vi "ControlPID_SeguidorLuz_2GL.vi"() -> ()   [LabVIEW 2015]
uses:
  <vilib>/MakerHub/LINX/Public/Peripherals/Digital/Digital Write N Chans.vi
  <vilib>/MakerHub/LINX/Public/Peripherals/Analog/Analog Read N Chans.vi
  <vilib>/MakerHub/LINX/Private/Local IO/LinxDigitalWrite.vi
  <vilib>/MakerHub/LINX/Public/Utilities/Check Channel.vi
  <vilib>/MakerHub/LINX/Private/Local IO/LinxAnalogRead.vi
  <vilib>/MakerHub/LINX/Public/Utilities/Open Serial.vi
  <vilib>/MakerHub/LINX/Private/Utilties/Generate Error.vi
  <vilib>/MakerHub/LINX/Public/Peripherals/PWM/PWM Set Duty Cycle N Chans.vi
  <vilib>/MakerHub/LINX/LMH-LINX.lvlib
  <vilib>/MakerHub/LINX/Public/Sensors/Distance/Ultrasonic/Ultrasonic.lvlib
panel:
  in  "Ajuste de\nTemp. °C":i32(slide)=63 scale=0.0..100.0
  out "Sistema \nActivo":bool
  out "PWM\nBase":dbl
  out "PWM\nPanel":dbl
  in  "Kp 2":dbl=1.5
  in  "Ki 2":dbl=0.001
  in  "Kd 2":dbl=0.001
  in  "Kd 1":dbl=0.001
  in  "Ki 1":dbl=0.001
  in  "Kp 1":dbl=1.0
  out "S. Luz 4":dbl format="%#_4g"
  out "S. Luz 3":dbl format="%#_4g"
  out "S. Luz 2":dbl format="%#_4g"
  out "S. Luz 1":dbl format="%#_4g"
  out "Bajo\nNivel":bool
  out "Baja\nTemp.":bool
  out "Temperatura °C":dbl(slide) scale=0.0..100.0
  out "Temperaturas °C":dbl[](array[numeric])=[29.0]
  out "Tanque L":dbl(slide) scale=0.0..1.0
  in  "Pausa":bool
  in  "Arranque":bool
  in  "Paro":bool
  out "Dispositivo conectado":string
  in  "Puerto":refnum<visa-resource-name>="COM3"
  # "Universidad Nacional Autónoma de México\nFacultad de Ingeniería\nLab. De Instrumentación Virtual\n\nProyecto Final: Calentador de agua mediante un seguidor solar"
  # "Configuración PID"
  # "Supervisión de sistema"
  # "Control de programa"
  # "Motor\nPanel"
  # "Motor\nBase"
  # "Saturación\nSensores"
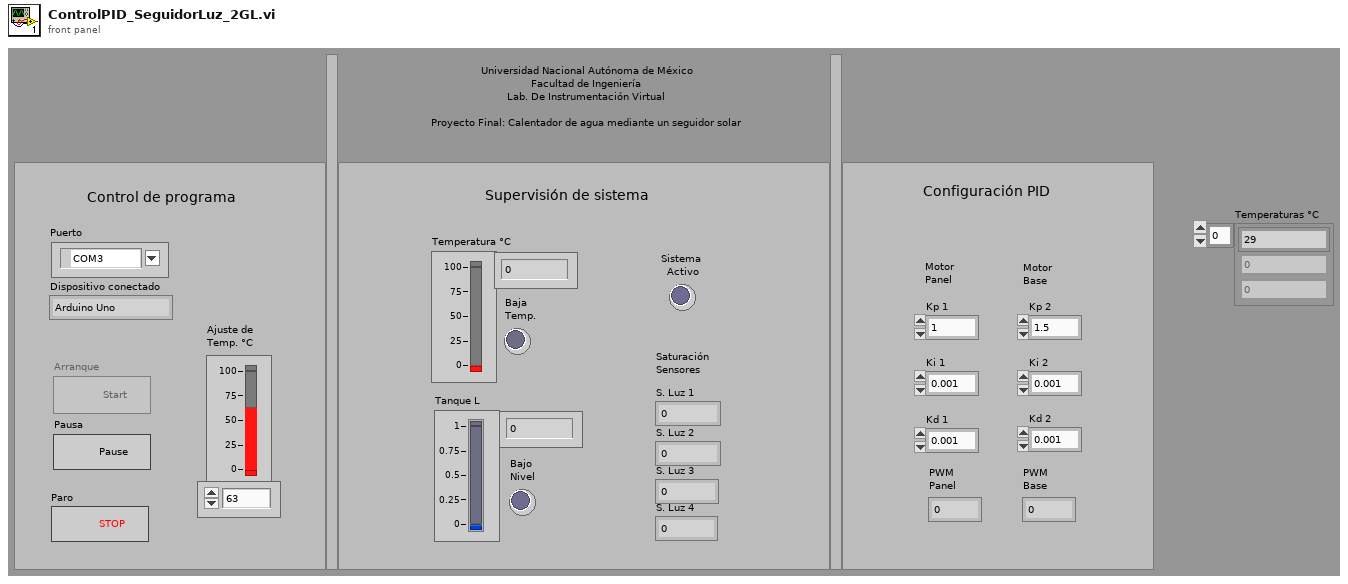
[diagram p1: front panel]
types:
  T1 = enum8{"Enabled", "Disabled", "Disabled and Grayed Out"}
  T2 = enum16{"Espera", "Nivel_Temp", "Reposo", "PID", "Fin"}
  T3 = typedef "LMH-LINX.lvlib/LINX Ref.ctl" = cluster{"IO":T4, "Interface":T5, "LINX Device Config":T6}
  T4 = typedef "LMH-LINX.lvlib/Platform.ctl" = enum16{"Remote", "Local"}
  T5 = typedef "LMH-LINX.lvlib/Interface.ctl" = enum16{"Serial", "TCP"}
  T6 = typedef "LMH-LINX.lvlib/Device.lvlib/LINX Device Config.ctl" = cluster{"Interface":T5, "COM Port":refnum<visa-resource-name>, "TCP Configuration":T7, "Device Family":u8, "Device ID":u8, "Device Name":string, "TCP Ref":refnum<k5>, "Channels":T8}
  T7 = typedef "LMH-LINX.lvlib/Device.lvlib/TCP Config.ctl" = cluster{"IP Address":string, "Port":u16}
  T8 = typedef "LMH-LINX.lvlib/Channels.ctl" = cluster{"DI":u8[], "DO":u8[], "AI":u8[], "AO":u8[], "PWM":u8[], "QE":u8[], "UART":u8[], "I2C 2":u8[], "SPI":u8[], "CAN":u8[], "Servo":u8[], "AI Ref (V)":dbl, "AI Resolution (Bits)":u8, "AO Ref (V)":dbl, "AO Resolution (Bits)":u8}
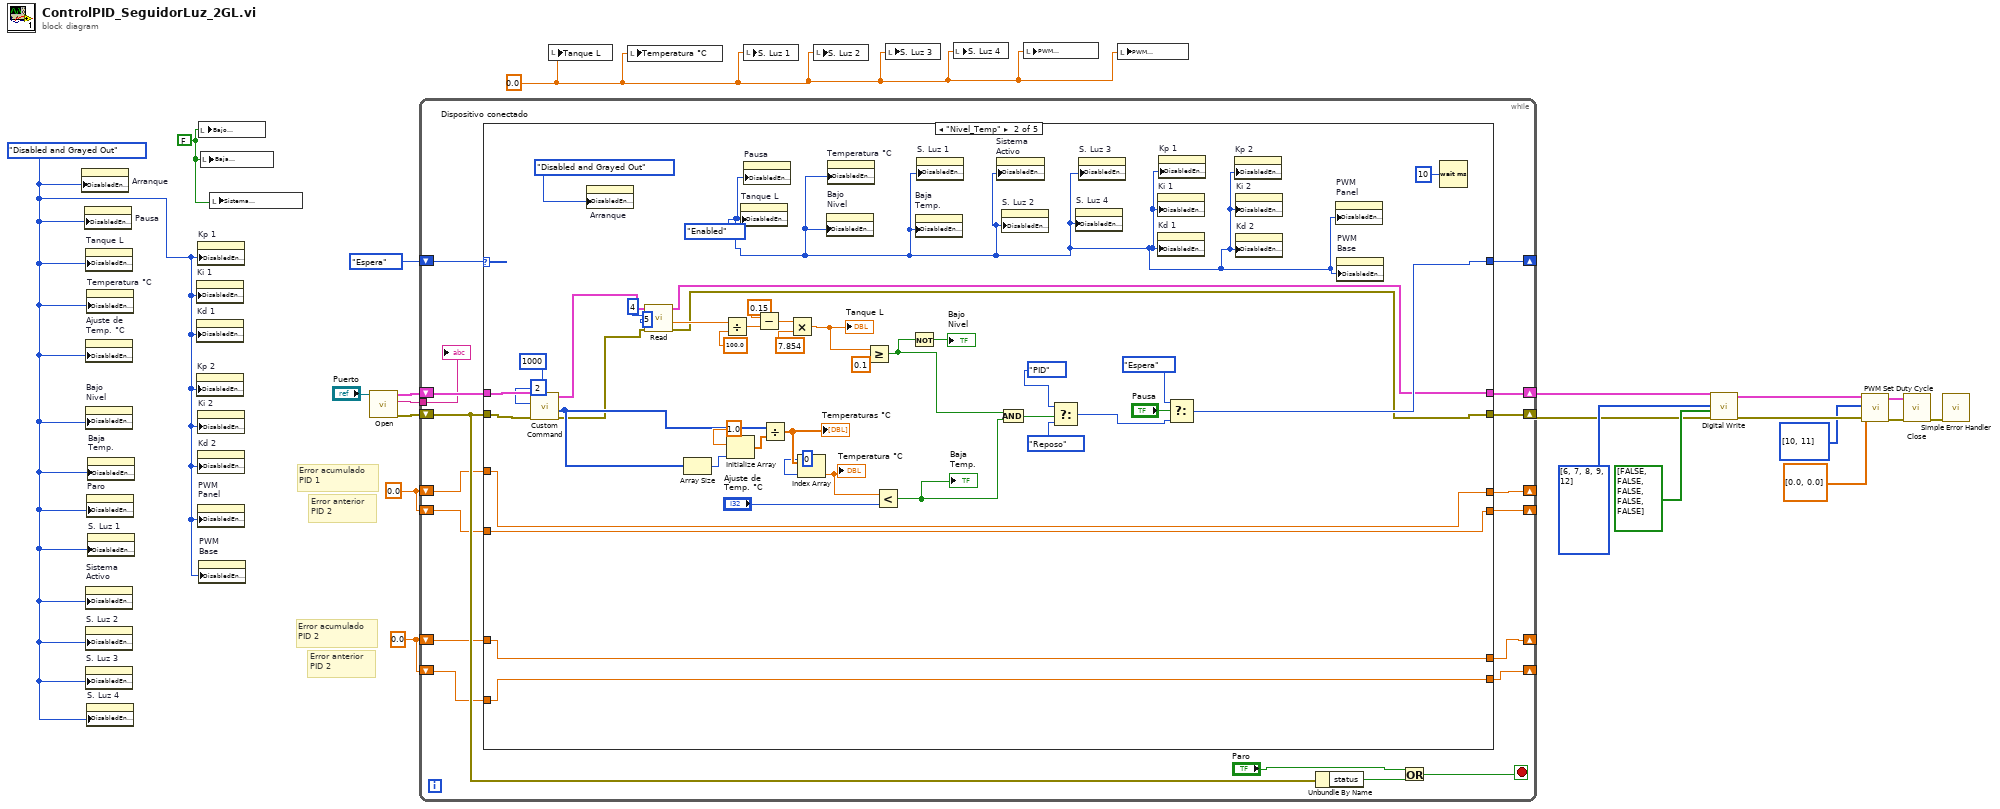
[diagram p0: block diagram]
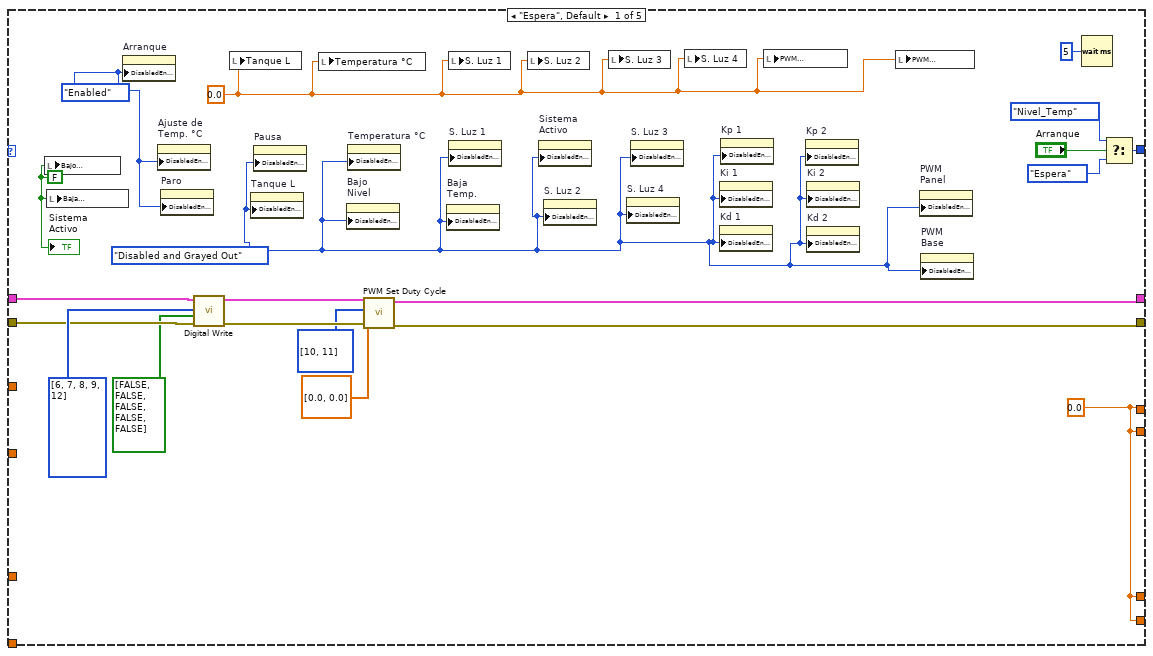
[diagram p2: hidden frame]
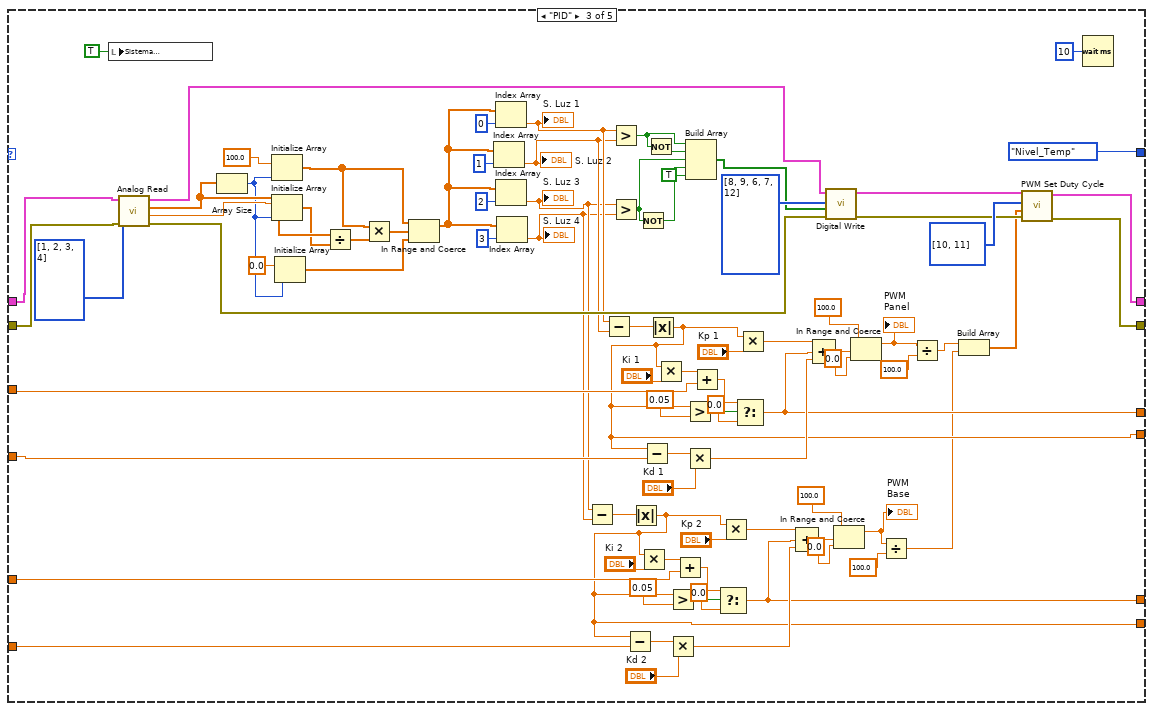
[diagram p3: hidden frame]
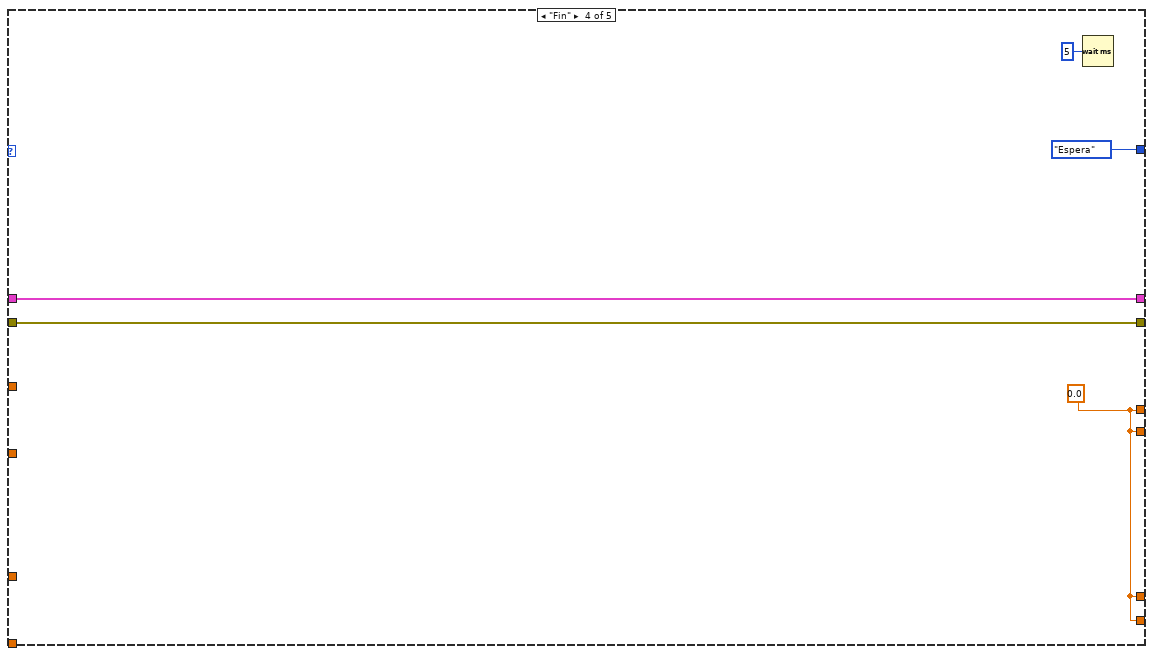
[diagram p4: hidden frame]
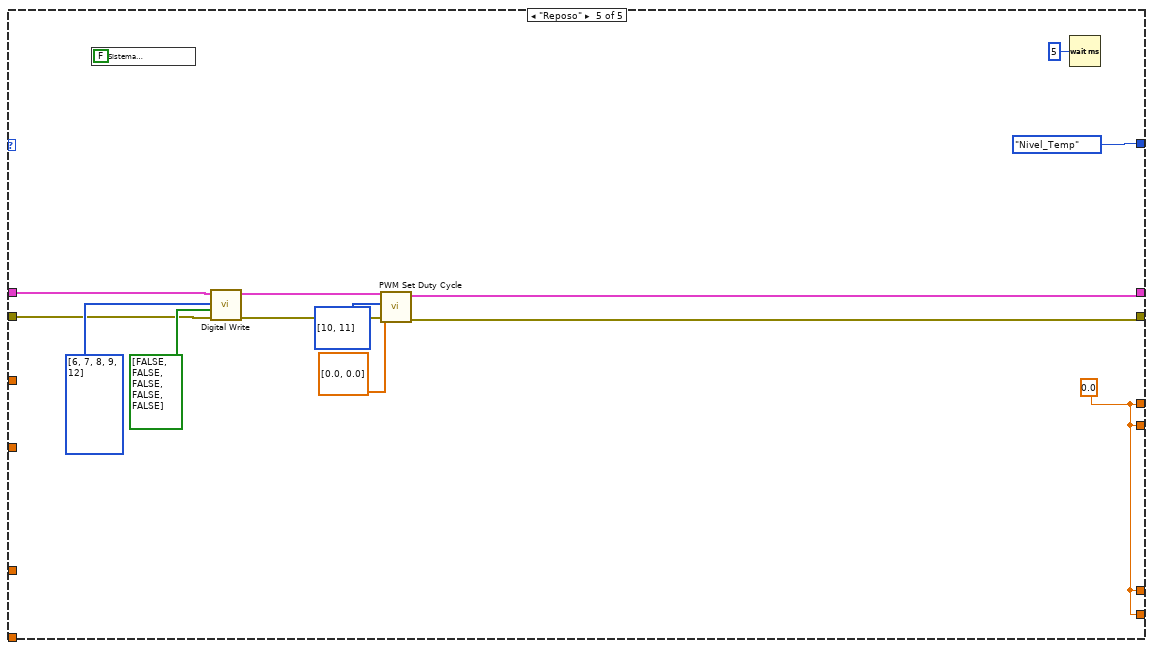
[diagram p5: hidden frame]
diagram:
  w11 = FALSE ("Bajo\nNivel")
  w13 = 0.0 ("Tanque L")
  w14 = 0.0
  w15 = 0.0
  w12 = T1."Disabled and Grayed Out" ("Disabled")
  # "Error anterior \nPID 2"
  # "Error acumulado\nPID 2"
  # "Error anterior \nPID 2"
  # "Error acumulado\nPID 1"
  n1 = property on="Arranque" class="Bool (strict)"("DisabledEnum"=w12) -> ()  [unwired: 2 in, 2 out]
  n2 = property on="Pausa" class="Bool (strict)"("DisabledEnum"=w12) -> ()  [unwired: 2 in, 2 out]
  n3 = property on="Tanque L" class="Slide (strict)"("DisabledEnum"=w12) -> ()  [unwired: 2 in, 2 out]
  n4 = property on="Ajuste de\nTemp. °C" class="Slide (strict)"("DisabledEnum"=w12) -> ()  [unwired: 2 in, 2 out]
  n5 = property on="Bajo\nNivel" class="Bool (strict)"("DisabledEnum"=w12) -> ()  [unwired: 2 in, 2 out]
  n6 = property on="Sistema \nActivo" class="Bool (strict)"("DisabledEnum"=w12) -> ()  [unwired: 2 in, 2 out]
  n7 = property on="S. Luz 2" class="DigNum (strict)"("DisabledEnum"=w12) -> ()  [unwired: 2 in, 2 out]
  n8 = property on="S. Luz 3" class="DigNum (strict)"("DisabledEnum"=w12) -> ()  [unwired: 2 in, 2 out]
  n9 = property on="Temperatura °C" class="Slide (strict)"("DisabledEnum"=w12) -> ()  [unwired: 2 in, 2 out]
  n10 = property on="Paro" class="Bool"("DisabledEnum"=w12) -> ()  [unwired: 2 in, 2 out]
  n11 = property on="S. Luz 4" class="DigNum (strict)"("DisabledEnum"=w12) -> ()  [unwired: 2 in, 2 out]
  n12 = property on="Baja\nTemp." class="Bool (strict)"("DisabledEnum"=w12) -> ()  [unwired: 2 in, 2 out]
  n13 = property on="S. Luz 1" class="DigNum (strict)"("DisabledEnum"=w12) -> ()  [unwired: 2 in, 2 out]
  n14 = property on="Ki 1" class="DigNum (strict)"("DisabledEnum"=w12) -> ()  [unwired: 2 in, 2 out]
  n15 = property on="Kd 1" class="DigNum (strict)"("DisabledEnum"=w12) -> ()  [unwired: 2 in, 2 out]
  n16 = property on="Kp 2" class="DigNum (strict)"("DisabledEnum"=w12) -> ()  [unwired: 2 in, 2 out]
  n17 = property on="Kp 1" class="DigNum (strict)"("DisabledEnum"=w12) -> ()  [unwired: 2 in, 2 out]
  n18 = property on="Ki 2" class="DigNum (strict)"("DisabledEnum"=w12) -> ()  [unwired: 2 in, 2 out]
  n19 = property on="Kd 2" class="DigNum (strict)"("DisabledEnum"=w12) -> ()  [unwired: 2 in, 2 out]
  n20 = property on="PWM\nPanel" class="DigNum (strict)"("DisabledEnum"=w12) -> ()  [unwired: 2 in, 2 out]
  n21 = local write "Bajo\nNivel"(w11) -> ()
  n22 = property on="PWM\nBase" class="DigNum (strict)"("DisabledEnum"=w12) -> ()  [unwired: 2 in, 2 out]
  n23 = local write "Baja\nTemp."(w11) -> ()
  n24 = local write "Sistema \nActivo"(w11) -> ()
  n25 = call-poly <vilib>:"Open.vi"("Serial Port"="Puerto") -> ("Error Out"=w17:errorcluster, "Device Name"=w18:string, "LINX Resource"=w19:T3)  [unwired: 8 in]
  n26 = while {
    shift-right: [w36] -> _
    shift-left: T2."Espera" -> [w39]
    tunnel: w18 -> [w37]
    shift-right: [w35] -> w2
    shift-left: w19 -> [w38]
    shift-right: [w34] -> w1
    shift-left: w17 -> [w33]
    shift-right: [w27] -> _
    shift-left: w15 -> [w29]
    shift-right: [w26] -> _
    shift-left: w15 -> [w28]
    shift-right: [w23] -> _
    shift-left: w14 -> [w25]
    shift-right: [w22] -> _
    shift-left: w14 -> [w24]
    stop <- w30 stop-if-true
    n27 = case shown="\"Nivel_Temp\"" w39 {
      tunnel: w38 -> [w54 w99 w141 w190 w199]
      tunnel: w33 -> [w53 w98 w140 w189 w198]
      tunnel: [w56 w74 T2."Nivel_Temp" T2."Espera" T2."Nivel_Temp"] -> w36
      tunnel: [w47 w68 w143 w190 w197] -> w35
      tunnel: [w46 w67 w142 w189 w196] -> w34
      tunnel: w29 -> [_ w66 w150 _ _]
      tunnel: w28 -> [_ w65 w144 _ _]
      tunnel: [w44 w66 w133 w187 w193] -> w27
      tunnel: [w44 w65 w132 w187 w193] -> w26
      tunnel: w25 -> [_ w64 w114 _ _]
      tunnel: w24 -> [_ w63 w113 _ _]
      tunnel: [w44 w64 w112 w187 w193] -> w23
      tunnel: [w44 w63 w111 w187 w193] -> w22
      frame "Espera", Default {
        w40 = T1."Disabled and Grayed Out" ("Disabled")
        w42 = 0.0 ("Tanque L")
        w43 = FALSE ("Bajo\nNivel")
        w44 = 0.0
        w41 = T1."Enabled" ("Disabled")
        n28 = local write "Bajo\nNivel"(w43) -> ()
        n29 = local write "Baja\nTemp."(w43) -> ()
        n30 = property on="Arranque" class="Bool (strict)"("DisabledEnum"=w41) -> ()  [unwired: 2 in, 2 out]
        n31 = property on="Ajuste de\nTemp. °C" class="Slide (strict)"("DisabledEnum"=w41) -> ()  [unwired: 2 in, 2 out]
        n32 = property on="Paro" class="Bool"("DisabledEnum"=w41) -> ()  [unwired: 2 in, 2 out]
        n33 = call-poly <vilib>:"Digital Write.vi"("Error In"=w53, "Values"=bool[] [FALSE, FALSE, FALSE, FALSE, FALSE], "DO Channels"=u8[] [6, 7, 8, 9, 12], "LINX Resource"=w54) -> ("Error Out"=w51:errorcluster, "LINX Resource"=w52:T3)  [unwired: 6 in]
        n34 = local write "Tanque L"(w42) -> ()
        n35 = property on="Tanque L" class="Slide (strict)"("DisabledEnum"=w40) -> ()  [unwired: 2 in, 2 out]
        n36 = property on="Pausa" class="Bool (strict)"("DisabledEnum"=w40) -> ()  [unwired: 2 in, 2 out]
        n37 = local write "Temperatura °C"(w42) -> ()
        n38 = property on="Bajo\nNivel" class="Bool (strict)"("DisabledEnum"=w40) -> ()  [unwired: 2 in, 2 out]
        n39 = property on="Temperatura °C" class="Slide (strict)"("DisabledEnum"=w40) -> ()  [unwired: 2 in, 2 out]
        n40 = call-poly <vilib>:"PWM Set Duty Cycle.vi"("Error In"=w51, "Duty Cycles"=dbl[] [0.0, 0.0], "PWM Channels"=u8[] [10, 11], "LINX Resource"=w52) -> ("Error Out"=w46:errorcluster, "LINX Resource"=w47:T3)  [unwired: 6 in]
        n41 = property on="Baja\nTemp." class="Bool (strict)"("DisabledEnum"=w40) -> ()  [unwired: 2 in, 2 out]
        n42 = local write "S. Luz 1"(w42) -> ()
        n43 = property on="S. Luz 1" class="DigNum (strict)"("DisabledEnum"=w40) -> ()  [unwired: 2 in, 2 out]
        n44 = local write "S. Luz 2"(w42) -> ()
        n45 = property on="Sistema \nActivo" class="Bool (strict)"("DisabledEnum"=w40) -> ()  [unwired: 2 in, 2 out]
        n46 = property on="S. Luz 2" class="DigNum (strict)"("DisabledEnum"=w40) -> ()  [unwired: 2 in, 2 out]
        n47 = local write "S. Luz 3"(w42) -> ()
        n48 = property on="S. Luz 4" class="DigNum (strict)"("DisabledEnum"=w40) -> ()  [unwired: 2 in, 2 out]
        n49 = property on="S. Luz 3" class="DigNum (strict)"("DisabledEnum"=w40) -> ()  [unwired: 2 in, 2 out]
        n50 = local write "S. Luz 4"(w42) -> ()
        n51 = property on="Ki 1" class="DigNum (strict)"("DisabledEnum"=w40) -> ()  [unwired: 2 in, 2 out]
        n52 = property on="Kd 1" class="DigNum (strict)"("DisabledEnum"=w40) -> ()  [unwired: 2 in, 2 out]
        n53 = property on="Kp 1" class="DigNum (strict)"("DisabledEnum"=w40) -> ()  [unwired: 2 in, 2 out]
        n54 = local write "PWM\nPanel"(w42) -> ()
        n55 = property on="Kp 2" class="DigNum (strict)"("DisabledEnum"=w40) -> ()  [unwired: 2 in, 2 out]
        n56 = property on="Ki 2" class="DigNum (strict)"("DisabledEnum"=w40) -> ()  [unwired: 2 in, 2 out]
        n57 = property on="Kd 2" class="DigNum (strict)"("DisabledEnum"=w40) -> ()  [unwired: 2 in, 2 out]
        n58 = local write "PWM\nBase"(w42) -> ()
        n59 = property on="PWM\nPanel" class="DigNum (strict)"("DisabledEnum"=w40) -> ()  [unwired: 2 in, 2 out]
        n60 = property on="PWM\nBase" class="DigNum (strict)"("DisabledEnum"=w40) -> ()  [unwired: 2 in, 2 out]
        n61 = Wait (ms)(milliseconds to wait=u32 5) -> ()  [unwired: 1 out]
        n62 = Select(t=T2."Nivel_Temp", s="Arranque", f=T2."Espera") -> (s? t:f=w56:T2)
        "Sistema \nActivo" <- w43
      }
      frame "Nivel_Temp" {
        w61 = T1."Enabled" ("Disabled")
        n63 = call <vilib>:"Custom Command.vi"("Timeout (100 ms)"=1000, "Error In"=w98, "Custom Command Number"=u16 2, "LINX Resource"=w99) -> ("Error Out"=w69:errorcluster, "Response"=w84:u8[], "LINX Resource"=w70:T3)  [unwired: 4 in, 1 out]
        n64 = property on="Arranque" class="Bool (strict)"("DisabledEnum"=T1."Disabled and Grayed Out" ("Disabled")) -> ()  [unwired: 2 in, 2 out]
        n65 = call <vilib>:"Read.vi"("Error In"=w69, "DO Channel"=u8 5, "DI Channel"=u8 4, "LINX Resource"=w70) -> ("Error Out"=w67:errorcluster, "Centimeters"=w92:dbl, "LINX Resource"=w68:T3)  [unwired: 4 in, 1 out]
        n66 = Array Size(array=w84) -> (size(s)=w95:i32)
        n67 = Divide(x=w92, y=100.0) -> (x/y=w90:dbl)
        n68 = Initialize Array(1.0 ("element"), w95) -> (w93:dbl[])
        n69 = property on="Tanque L" class="Slide (strict)"("DisabledEnum"=w61) -> ()  [unwired: 2 in, 2 out]
        n70 = property on="Pausa" class="Bool (strict)"("DisabledEnum"=w61) -> ()  [unwired: 2 in, 2 out]
        n71 = Subtract(x=0.15, y=w90) -> (x-y=w88:dbl)
        n72 = Divide(x=w84, y=w93) -> (x/y=w83:dbl[])
        "Temperaturas °C" <- w83
        n73 = Multiply(x=w88, y=7.854) -> (x*y=w86:dbl)
        "Tanque L" <- w86
        n74 = Index Array(array=w83, index=0) -> (element=w81:dbl)
        "Temperatura °C" <- w81
        n75 = property on="Bajo\nNivel" class="Bool (strict)"("DisabledEnum"=w61) -> ()  [unwired: 2 in, 2 out]
        n76 = property on="Temperatura °C" class="Slide (strict)"("DisabledEnum"=w61) -> ()  [unwired: 2 in, 2 out]
        n77 = Greater Or Equal?(x=w86, y=0.1) -> (x >= y?=w60:bool)
        n78 = Less?(x=w81, y="Ajuste de\nTemp. °C") -> (x < y?=w72:bool)
        "Baja\nTemp." <- w72
        n79 = Not(x=w60) -> (.not. x?=→"Bajo\nNivel":bool)
        n80 = property on="Baja\nTemp." class="Bool (strict)"("DisabledEnum"=w61) -> ()  [unwired: 2 in, 2 out]
        n81 = property on="S. Luz 1" class="DigNum (strict)"("DisabledEnum"=w61) -> ()  [unwired: 2 in, 2 out]
        n82 = property on="Sistema \nActivo" class="Bool (strict)"("DisabledEnum"=w61) -> ()  [unwired: 2 in, 2 out]
        n83 = And(x=w60, y=w72) -> (x .and. y?=w80:bool)
        n84 = property on="S. Luz 2" class="DigNum (strict)"("DisabledEnum"=w61) -> ()  [unwired: 2 in, 2 out]
        n85 = Select(t=T2."PID", s=w80, f=T2."Reposo") -> (s? t:f=w76:T2)
        n86 = property on="S. Luz 4" class="DigNum (strict)"("DisabledEnum"=w61) -> ()  [unwired: 2 in, 2 out]
        n87 = property on="S. Luz 3" class="DigNum (strict)"("DisabledEnum"=w61) -> ()  [unwired: 2 in, 2 out]
        n88 = property on="Ki 1" class="DigNum (strict)"("DisabledEnum"=w61) -> ()  [unwired: 2 in, 2 out]
        n89 = property on="Kd 1" class="DigNum (strict)"("DisabledEnum"=w61) -> ()  [unwired: 2 in, 2 out]
        n90 = property on="Kp 1" class="DigNum (strict)"("DisabledEnum"=w61) -> ()  [unwired: 2 in, 2 out]
        n91 = Select(t=T2."Espera", s="Pausa", f=w76) -> (s? t:f=w74:T2)
        n92 = property on="Kp 2" class="DigNum (strict)"("DisabledEnum"=w61) -> ()  [unwired: 2 in, 2 out]
        n93 = property on="Ki 2" class="DigNum (strict)"("DisabledEnum"=w61) -> ()  [unwired: 2 in, 2 out]
        n94 = property on="Kd 2" class="DigNum (strict)"("DisabledEnum"=w61) -> ()  [unwired: 2 in, 2 out]
        n95 = property on="PWM\nPanel" class="DigNum (strict)"("DisabledEnum"=w61) -> ()  [unwired: 2 in, 2 out]
        n96 = property on="PWM\nBase" class="DigNum (strict)"("DisabledEnum"=w61) -> ()  [unwired: 2 in, 2 out]
        n97 = Wait (ms)(milliseconds to wait=u32 10) -> ()  [unwired: 1 out]
      }
      frame "PID" {
        n98 = local write "Sistema \nActivo"(TRUE ("Sistema \nActivo")) -> ()
        n99 = call-poly <vilib>:"Analog Read.vi"("Error In"=w140, "AI Channel(s)"=u8[] [1, 2, 3, 4], "LINX Resource"=w141) -> ("Error Out"=w165:errorcluster, "AI Ref"=w184:dbl, "Voltages"=w183:dbl[], "LINX Resource"=w166:T3)  [unwired: 5 in]
        n100 = Array Size(array=w183) -> (size(s)=w178:i32)
        n101 = Initialize Array(100.0 ("element"), w178) -> (w179:dbl[])
        n102 = Initialize Array(w184, w178) -> (w182:dbl[])
        n103 = Initialize Array(0.0 ("element"), w178) -> (w176:dbl[])
        n104 = Divide(x=w183, y=w182) -> (x/y=w181:dbl[])
        n105 = Multiply(x=w179, y=w181) -> (x*y=w180:dbl[])
        n106 = In Range and Coerce(upper limit=w179, x=w180, lower limit=w176) -> (coerced(x)=w171:dbl[])  [unwired: 1 out]
        n107 = Index Array(array=w171, index=1) -> (element=w155:dbl)
        "S. Luz 2" <- w155
        n108 = Index Array(array=w171, index=0) -> (element=w156:dbl)
        "S. Luz 1" <- w156
        n109 = Index Array(array=w171, index=2) -> (element=w116:dbl)
        "S. Luz 3" <- w116
        n110 = Index Array(array=w171, index=3) -> (element=w115:dbl)
        "S. Luz 4" <- w115
        n111 = Subtract(x=w116, y=w115) -> (x-y=w118:dbl)
        n112 = Subtract(x=w156, y=w155) -> (x-y=w153:dbl)
        n113 = Greater?(x=w156, y=w155) -> (0:w162:bool)
        n114 = Greater?(x=w116, y=w115) -> (0:w161:bool)
        n115 = Absolute Value(x=w118) -> (abs(x)=w111:dbl)
        n116 = Subtract(x=w111, y=w113) -> (x-y=w126:dbl)
        n117 = Not(x=w161) -> (.not. x?=w160:bool)
        n118 = Multiply(x=w111, y="Ki 2") -> (x*y=w120:dbl)
        n119 = Not(x=w162) -> (.not. x?=w163:bool)
        n120 = Absolute Value(x=w153) -> (abs(x)=w132:dbl)
        n121 = Subtract(x=w132, y=w144) -> (x-y=w139:dbl)
        n122 = Multiply(x=w132, y="Ki 1") -> (x*y=w151:dbl)
        n123 = Greater?(x=w111, y=0.05) -> (0:w123:bool)
        n124 = Multiply(x=w126, y="Kd 2") -> (x*y=w128:dbl)
        n125 = Add(x=w120, y=w114) -> (x+y=w121:dbl)
        n126 = Greater?(x=w132, y=0.05) -> (0:w147:bool)
        n127 = Multiply(x=w139, y="Kd 1") -> (x*y=w137:dbl)
        n128 = Build Array(w162, w163, w161, w160, TRUE ("element")) -> (w158:bool[])
        n129 = Add(x=w151, y=w150) -> (x+y=w149:dbl)
        n130 = Select(t=w121, s=w123, f=0.0) -> (s? t:f=w112:dbl)
        n131 = Multiply(x=w111, y="Kp 2") -> (x*y=w125:dbl)
        n132 = Select(t=w149, s=w147, f=0.0) -> (s? t:f=w133:dbl)
        n133 = Multiply(x=w132, y="Kp 1") -> (x*y=w145:dbl)
        n134 = Compound Arithmetic op=ADD(w125, w112, w128) -> (w131:dbl)
        n135 = Compound Arithmetic op=ADD(w145, w133, w137) -> (w134:dbl)
        n136 = call-poly <vilib>:"Digital Write.vi"("Error In"=w165, "Values"=w158, "DO Channels"=u8[] [8, 9, 6, 7, 12], "LINX Resource"=w166) -> ("Error Out"=w169:errorcluster, "LINX Resource"=w168:T3)  [unwired: 6 in]
        n137 = In Range and Coerce(upper limit=100.0, x=w131, lower limit=0.0) -> (coerced(x)=w106:dbl)  [unwired: 1 out]
        "PWM\nBase" <- w106
        n138 = In Range and Coerce(upper limit=100.0, x=w134, lower limit=0.0) -> (coerced(x)=w109:dbl)  [unwired: 1 out]
        "PWM\nPanel" <- w109
        n139 = Divide(x=w106, y=100.0) -> (x/y=w104:dbl)
        n140 = Divide(x=w109, y=100.0) -> (x/y=w105:dbl)
        n141 = Build Array(w105, w104) -> (w103:dbl[])
        n142 = call-poly <vilib>:"PWM Set Duty Cycle.vi"("Error In"=w169, "Duty Cycles"=w103, "PWM Channels"=u8[] [10, 11], "LINX Resource"=w168) -> ("Error Out"=w142:errorcluster, "LINX Resource"=w143:T3)  [unwired: 6 in]
        n143 = Wait (ms)(milliseconds to wait=u32 10) -> ()  [unwired: 1 out]
      }
      frame "Fin" {
        w187 = 0.0
        n144 = Wait (ms)(milliseconds to wait=u32 5) -> ()  [unwired: 1 out]
      }
      frame "Reposo" {
        w193 = 0.0
        n145 = local write "Sistema \nActivo"(FALSE ("Sistema \nActivo")) -> ()
        n146 = call-poly <vilib>:"Digital Write.vi"("Error In"=w198, "Values"=bool[] [FALSE, FALSE, FALSE, FALSE, FALSE], "DO Channels"=u8[] [6, 7, 8, 9, 12], "LINX Resource"=w199) -> ("Error Out"=w203:errorcluster, "LINX Resource"=w204:T3)  [unwired: 6 in]
        n147 = call-poly <vilib>:"PWM Set Duty Cycle.vi"("Error In"=w203, "Duty Cycles"=dbl[] [0.0, 0.0], "PWM Channels"=u8[] [10, 11], "LINX Resource"=w204) -> ("Error Out"=w196:errorcluster, "LINX Resource"=w197:T3)  [unwired: 6 in]
        n148 = Wait (ms)(milliseconds to wait=u32 5) -> ()  [unwired: 1 out]
      }
    }
    n149 = Unbundle By Name(w33) -> ("status"=w31:bool)
    n150 = Or(x="Paro", y=w31) -> (x .or. y?=w30:bool)
    "Dispositivo conectado" <- w37
  }
  n151 = local write "Tanque L"(w13) -> ()
  n152 = local write "Temperatura °C"(w13) -> ()
  n153 = local write "S. Luz 1"(w13) -> ()
  n154 = local write "S. Luz 2"(w13) -> ()
  n155 = local write "S. Luz 3"(w13) -> ()
  n156 = local write "S. Luz 4"(w13) -> ()
  n157 = local write "PWM\nPanel"(w13) -> ()
  n158 = local write "PWM\nBase"(w13) -> ()
  n159 = call-poly <vilib>:"Digital Write.vi"("Error In"=w1, "Values"=bool[] [FALSE, FALSE, FALSE, FALSE, FALSE], "DO Channels"=u8[] [6, 7, 8, 9, 12], "LINX Resource"=w2) -> ("Error Out"=w8:errorcluster, "LINX Resource"=w9:T3)  [unwired: 6 in]
  n160 = call-poly <vilib>:"PWM Set Duty Cycle.vi"("Error In"=w8, "Duty Cycles"=dbl[] [0.0, 0.0], "PWM Channels"=u8[] [10, 11], "LINX Resource"=w9) -> ("Error Out"=w3:errorcluster, "LINX Resource"=w4:T3)  [unwired: 6 in]
  n161 = call <vilib>:"Close.vi"("Error In"=w3, "LINX Resource"=w4) -> ("Error Out"=w16:errorcluster)  [unwired: 9 in]
  n162 = call <vilib>:"Simple Error Handler.vi"("error in (no error)"=w16) -> ()  [unwired: 4 in, 5 out]
